vi "gaussian_fit.vi"() -> ()   [LabVIEW 2018]
panel:
  out "abs(x)":dbl
  out "Array":dbl[](array[numeric]) caption="数组"
  out "XY图":cluster{"all rows":dbl[], "Array":dbl[]}[](graph)
  in  "file path (dialog if empty)":path caption="文件路径 （空时为对话框）"
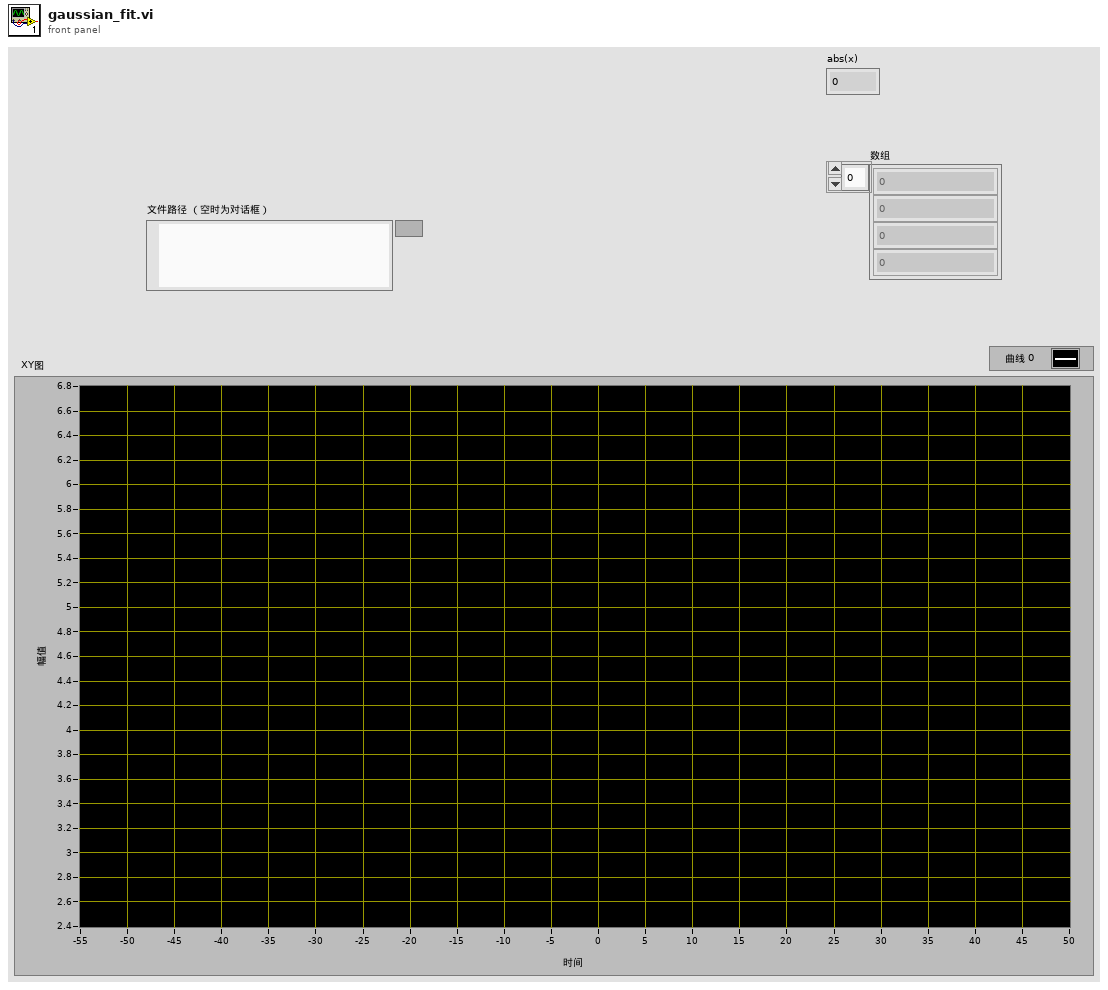
[diagram p1: front panel]
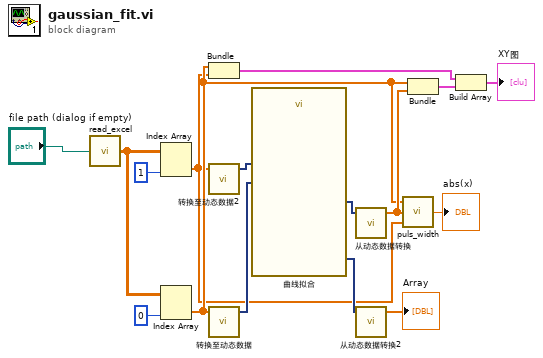
[diagram p0: block diagram]
diagram:
  n1 = call "read_excel.vi"("file path (dialog if empty)"="file path (dialog if empty)") -> ("data_out"=w5:dbl[][])
  n2 = Index Array(array=w5, index (col)=1 ("禁用的索引 (列)")) -> (element=w1:dbl[])  [unwired: 1 in]
  n3 = Index Array(array=w5, index (col)=0 ("禁用的索引 (列)")) -> (element=w3:dbl[])  [unwired: 1 in]
  n4 = Bundle("data_out"=w3, "data_out"=w1) -> (w11:cluster{"data_out":dbl[], "data_out":dbl[]})  [unwired: 1 in]
  n5 = call "转换至动态数据2"("Array"=w1) -> ("Dynamic Data Type"=w13:dynamicdata)  [unwired: 3 in]
  n6 = call "转换至动态数据"("Array"=w3) -> ("Dynamic Data Type"=w14:dynamicdata)  [unwired: 3 in]
  n7 = call "曲线拟合"("Locations"=w14, "Signals"=w13) -> ("best fit"=w12:dynamicdata, "non-linear coefficients"=w8:dynamicdata)  [unwired: 5 in, 3 out]
  n8 = call "从动态数据转换"("Dynamic Data Type"=w12) -> ("Array"=w4:dbl[])  [unwired: 3 in]
  n9 = call "从动态数据转换2"("Dynamic Data Type"=w8) -> ("Array"=→"Array":dbl[])  [unwired: 3 in]
  n10 = call "puls_width.vi"("Y0"=w1, "Y"=w4, "X"=w3) -> ("abs(x)"=→"abs(x)":dbl)
  n11 = Bundle("data_out"=w3, "Array"=w4) -> (w10:cluster{"data_out":dbl[], "Array":dbl[]})  [unwired: 1 in]
  n12 = Build Array(w11, w10) -> (→"XY图":cluster{"data_out":dbl[], "Array":dbl[]}[])
